vi "Create New Test Executive.vi"(8 "error in (no error)":errorcluster, 9 "Linked List ID":string, 10 "Name":string, 11 "Test Executive in":refnum<class "Test Executive.lvclass">) -> (0 "error out":errorcluster, 3 "Test Executive out":refnum<class "Test Executive.lvclass">, 5 "Test Executive ID out":string)   [LabVIEW 2019, in "Test Executive.lvlib" / "Test Executive.lvclass"]
uses:
  <vilib>/gpm_packages/@cs/test-executive/Source/Test Executive/TestExecutive/Test Executive.lvclass
  <vilib>/gpm_packages/@cs/linked-list/Source/Linked List/Linked List/Linked List.lvclass
  C:/Program Files/National Instruments/LabVIEW 2019/vi.lib/gpm_packages/@cs/linked-list/Source/Linked List/ILinkedList/ILinked List.lvclass
  <vilib>/gpm_packages/@cs/test-executive/Source/Test Executive/TestExecutive/Test Executive.lvclass/Test Executive.ctl
  <vilib>/gpm_packages/@cs/linked-list/Source/Linked List/Linked List Ref/Linked List Ref.lvclass
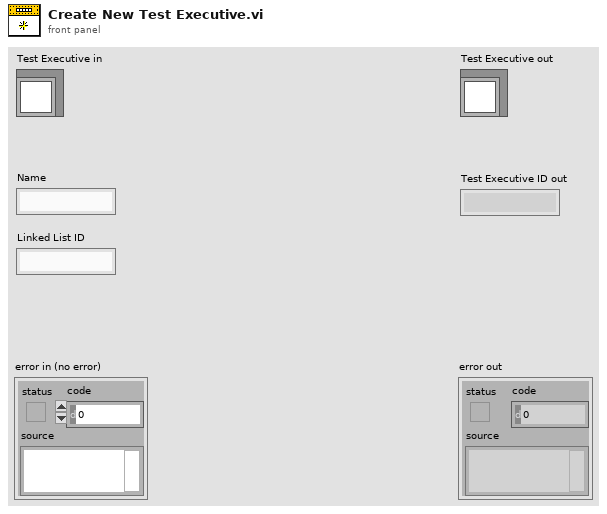
[diagram p1: front panel]
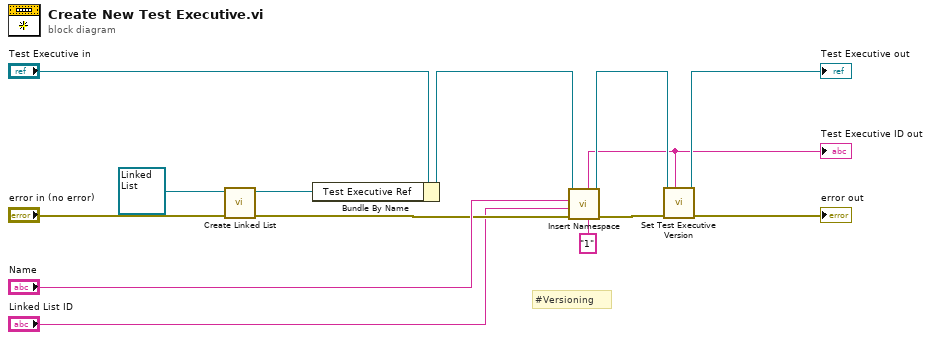
[diagram p0: block diagram]
diagram:
  # "#Versioning"
  n1 = call <vilib>:"Create Linked List.vi"("error in (no error)"="error in (no error)", "Linked List"=refnum<class "Linked List.lvclass"> refnum ("Linked Lists.lvlib:Linked List.lvclass")) -> ("error out"=w8:errorcluster, "Linked List Ref"=w11:refnum<data-value>)  [unwired: 8 in]
  n2 = Bundle By Name(cluster="Test Executive in", "Test Executive Ref"=w11) -> (w9:refnum<class "Test Executive.lvclass">)
  n3 = call-dynamic "Insert Namespace.vi"("Test File Version Number"="1" ("File Version Number"), "error in (no error)"=w8, "Linked List ID"="Linked List ID", "Name"="Name", "Test Executive in"=w9) -> ("error out"=w5:errorcluster, "Test Executive out"=w3:refnum<class "Test Executive.lvclass">, "Unique ID out"=w1:string)  [unwired: 3 in, 1 out]
  "Test Executive ID out" <- w1
  n4 = call-dynamic "Set Test Executive Version.vi"("Unique ID"=w1, "error in (no error)"=w5, "Test Executive in"=w3) -> ("error out"=→"error out":errorcluster, "Test Executive out"=→"Test Executive out":refnum<class "Test Executive.lvclass">)  [unwired: 7 in]
